vi "test2.vi"() -> ()   [LabVIEW 2020]
panel:
  out "sortie d'erreur":errorcluster
  in  "entrée d'erreur (pas d'erreur)":errorcluster
  in  "Nom de ressource VISA":refnum<visa-resource-name>
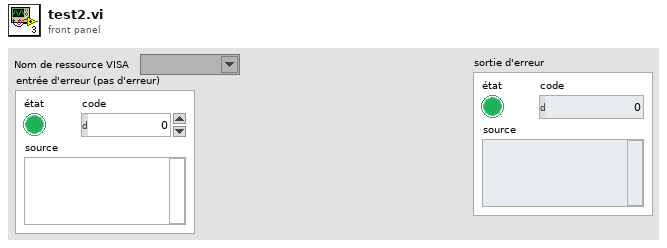
[diagram p1: front panel]
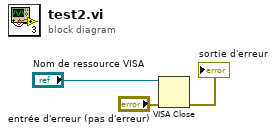
[diagram p0: block diagram]
diagram:
  n1 = VISA Close(VISA resource name="Nom de ressource VISA", error in (no error)="entrée d'erreur (pas d'erreur)") -> (error out=→"sortie d'erreur":errorcluster)
